vi "Write WorkTable.vi"(8 "error in (no error)":errorcluster, 10 "FlexWorktable":refnum<class "FlexWorktable.lvclass">, 11 "Gantry Class in":refnum<class "Gantry.lvclass">) -> (0 "error out":errorcluster, 3 "Gantry Class out":refnum<class "Gantry.lvclass">)   [LabVIEW 2024, in "Gantry.lvclass"]
uses:
  Gantry.lvclass
  FlexWorktable/FlexWorktable.lvclass
  Gantry.lvclass/Gantry.ctl
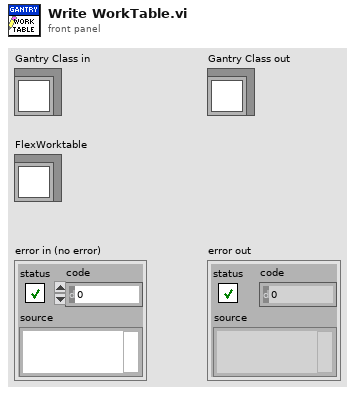
[diagram p1: front panel]
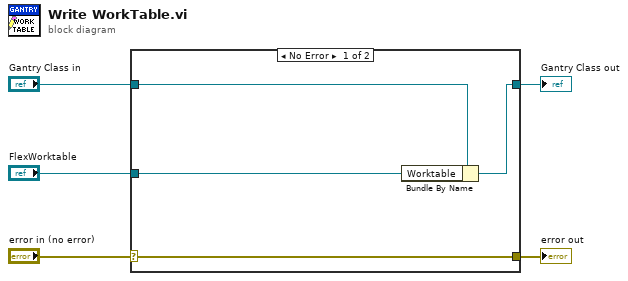
[diagram p0: block diagram]
diagram:
  n1 = case shown="No Error" "error in (no error)" {
    selector: "error in (no error)" -> [w9 w10]
    tunnel: [w9 w10] -> w4
    tunnel: [w7 w11] -> w2
    tunnel: "Gantry Class in" -> [w8 w11]
    tunnel: "FlexWorktable" -> [w6 _]
    frame No Error {
      n2 = Bundle By Name(cluster=w8, "Worktable"=w6) -> (w7:refnum<class "Gantry.lvclass">)
    }
    frame Error {
    }
  }
  "error out" <- w4
  "Gantry Class out" <- w2
